vi "2D X&Y Commands.vi"(6 "Kill X&Y waves?":bool=TRUE, 8 "error in (no error)":errorcluster, 9 "Y wave":string, 10 "X wave":string, 11 "2D wave":string) -> (0 "error out":errorcluster, 3 "result string":string)   [LabVIEW 2016, in "LVtoITX.lvclass"]
uses:
  LVtoITX.lvclass
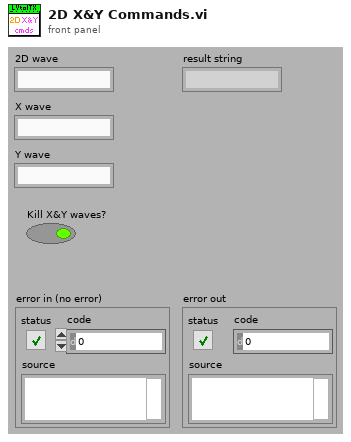
[diagram p1: front panel]
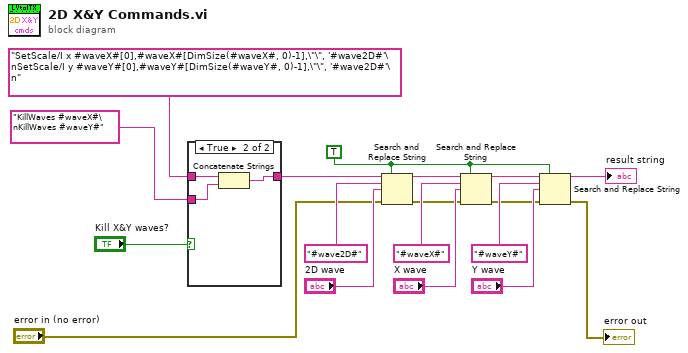
[diagram p0: block diagram]
diagram:
  w14 = TRUE ("replace all? (F)")
  n1 = case shown="True" "Kill X&Y waves?" {
    tunnel: "SetScale/I x #waveX#[0],#waveX#[DimSize(#waveX#, 0)-1],\"\", '#wave2D#'\nSetScale/I y #waveY#[0],#waveY#[DimSize(#waveY#, 0)-1],\"\", '#wave2D#'\n" ("input string 1") -> [w19 w22]
    tunnel: [w19 w21] -> w7
    tunnel: "KillWaves #waveX#\nKillWaves #waveY#" ("input string 2") -> [_ w20]
    frame False {
    }
    frame True {
      n2 = Concatenate Strings(w22, w20) -> (w21:string)
    }
  }
  n3 = Search and Replace String(replace all?=w14, input string=w7, search string="#wave2D#", replace string="2D wave", error in="error in (no error)") -> (result string=w9:string, error out=w3:errorcluster)  [unwired: 5 out]
  n4 = Search and Replace String(replace all?=w14, input string=w9, search string="#waveX#", replace string="X wave", error in=w3) -> (result string=w11:string, error out=w2:errorcluster)  [unwired: 5 out]
  n5 = Search and Replace String(replace all?=w14, input string=w11, search string="#waveY#", replace string="Y wave", error in=w2) -> (result string=→"result string":string, error out=→"error out":errorcluster)  [unwired: 5 out]
